vi "Receiver Test.vi"() -> ()   [LabVIEW 2012]
panel:
  out "Image":T1(plugin-control)
  in  "stop":bool
  in  "IP Address":string="127.0.0.1"
  in  "Port":i32=58432
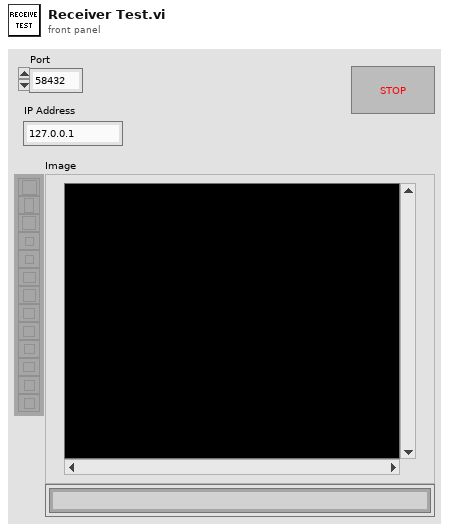
[diagram p1: front panel]
types:
  T1 = typedef "IMAQ Image.ctl" = refnum<image>
  T2 = typedef "Image Type" = u32
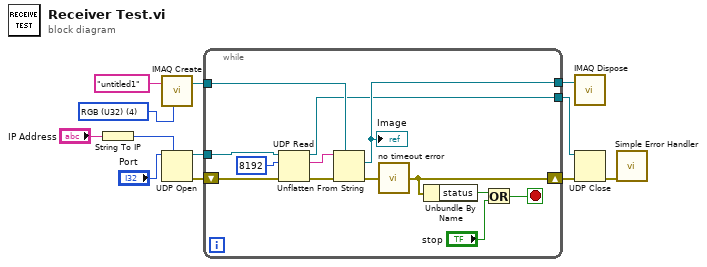
[diagram p0: block diagram]
diagram:
  w2 = T2 4 items=["Grayscale (U8)", "Grayscale (I16)", "Grayscale (SGL)", "Complex (CSG)", "RGB (U32)", "HSL (U32)", "RGB (U64)", "Grayscale (U16)"] ("Image Type")
  n1 = String To IP(1:"IP Address") -> (0:w1:u32)
  n2 = call "IMAQ Create"("Image Name"="untitled1", "Image Type"=w2) -> ("New Image"=w4:T1)  [unwired: 3 in, 1 out]
  n3 = UDP Open(7:w1, 11:"Port") -> (port=w12:refnum<k16>, 0:w10:errorcluster)  [unwired: 3 in, 1 out]
  n4 = while {
    tunnel: w12 -> [w25]
    tunnel: [w13] -> w11
    shift-right: [w20] -> w6
    shift-left: w10 -> [w21]
    tunnel: w4 -> [w16]
    tunnel: [w15] -> w3
    stop <- w22 stop-if-true
    n5 = UDP Read(connection ID=w25, max size (548)=8192, 8:w21) -> (data out=w19:string, error out=w17:errorcluster, 3:w13:refnum<k16>)  [unwired: 1 in, 2 out]
    n6 = Unflatten From String(type=w16, binary string=w19, error in (no error)=w17) -> (value=w15:T1, error out=w14:errorcluster)  [unwired: 2 in, 1 out]
    "Image" <- w15
    n7 = call "no timeout error.vi"("error in (no error)"=w14) -> ("error out"=w20:errorcluster)
    n8 = Unbundle By Name(w20) -> ("status"=w24:bool)
    n9 = Or(x=w24, y="stop") -> (x .or. y?=w22:bool)
  }
  n10 = call "IMAQ Dispose"("Image"=w3) -> ()  [unwired: 5 in, 1 out]
  n11 = UDP Close(connection ID=w11, 8:w6) -> (error out=w8:errorcluster)  [unwired: 1 out]
  n12 = call <vilib>:"Simple Error Handler.vi"("error in (no error)"=w8) -> ()  [unwired: 1 in, 8 out]
